vi "DELETE_req_PS.vi"(7 "Headers":string, 8 "error in":errorcluster, 11 "URL":string) -> (0 "error out":errorcluster, 3 "DELETE Request":string)   [LabVIEW 2016, in "Request.lvclass"]
uses:
  Request.lvclass
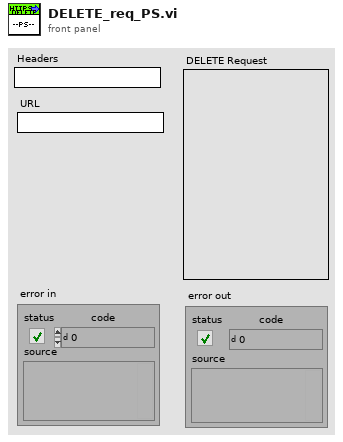
[diagram p1: front panel]
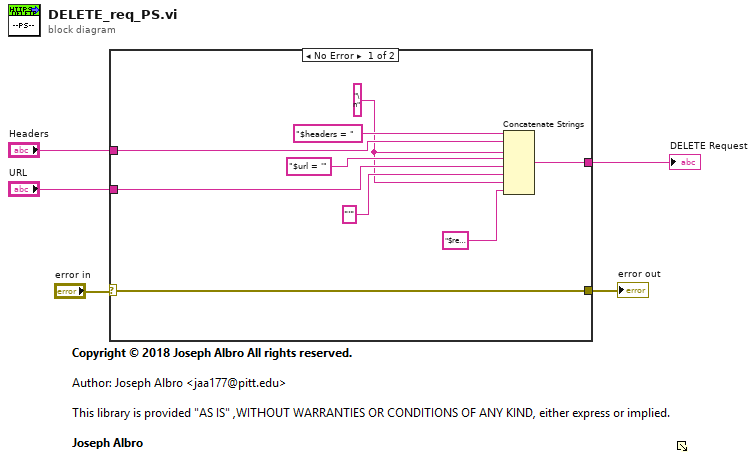
[diagram p0: block diagram]
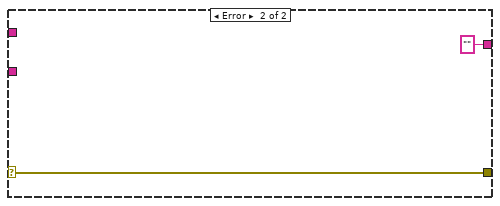
[diagram p2: hidden frame]
diagram:
  n1 = case shown="No Error" "error in" {
    selector: "error in" -> [w7 w15]
    tunnel: "Headers" -> [w14 _]
    tunnel: "URL" -> [w11 _]
    tunnel: [w9 ""] -> w3
    tunnel: [w7 w15] -> w1
    frame No Error {
      w8 = "\n"
      n2 = Concatenate Strings("$headers = ", w14, w8, "$url = '" ("string"), w11, "'" ("string"), w8, "$request = \ntry { \nInvoke-WebRequest -Method 'DELETE' -uri $url -Headers $headers \n$err = 'false' \n} catch { \n    $_.exception\n    $errorresponse = $error[0].errordetails.message\n    $err = 'true'\n    $errorresponse\n}\nif ($err -eq 'false') {\n    $request.rawcontent\n} else {\n    $request\n}" ("string")) -> (w9:string)
    }
    frame Error {
    }
  }
  "DELETE Request" <- w3
  "error out" <- w1
